vi "Parse Message.vi"   [LabVIEW 2012, in "MicroStrain 3DM-GXx.lvlib"]
doc: "Polymorphic VI used to parse the various message types received by the device into useable values."
uses:
  <instrlib>/MicroStrain 3DM-GXx/MicroStrain 3DM-GXx.lvlib
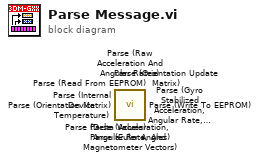
[diagram p0: block diagram]
diagram:
  n1 = call <instrlib>:"Parse (Acceleration, Angular Rate, And Magnetometer Vectors).vi"() -> ()  [unwired: 12 in, 4 out]
  n2 = call <instrlib>:"Parse (Orientation Update Matrix).vi"() -> ()  [unwired: 14 in, 2 out]
  n3 = call <instrlib>:"Parse (Orientation Matrix).vi"() -> ()  [unwired: 14 in, 2 out]
  n4 = call <instrlib>:"Parse (Write To EEPROM).vi"() -> ()  [unwired: 15 in, 1 out]
  n5 = call <instrlib>:"Parse (Read From EEPROM).vi"() -> ()  [unwired: 15 in, 1 out]
  n6 = call <instrlib>:"Parse (Raw Acceleration And Angular Rates).vi"() -> ()  [unwired: 13 in, 3 out]
  n7 = call <instrlib>:"Parse (Internal Device Temperature).vi"() -> ()  [unwired: 14 in, 2 out]
  n8 = call <instrlib>:"Parse (Gyro Stabilized Acceleration, Angular Rate, And Magnetometer Vectors).vi"() -> ()  [unwired: 12 in, 4 out]
  n9 = call <instrlib>:"Parse (Delta Values).vi"() -> ()  [unwired: 13 in, 3 out]
  n10 = call <instrlib>:"Parse (Euler Angles).vi"() -> ()  [unwired: 12 in, 4 out]
